vi "Calculator_Calculator-teardown.vi"(10 "Numeric":i32, 11 "test case ID":string) -> (3 "result":bool)   [LabVIEW 2020]
doc: "The teardown VI should be executed after the VI under test in the harness VI. In this VI you can evaluate the outputs of the VI under test.\n\nSee the Help Document for more information. (<b>Help</b> > <b>InstaCoverage Help...</b>)"
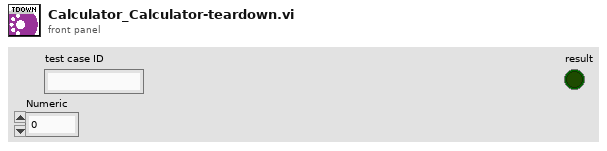
[diagram p1: front panel]
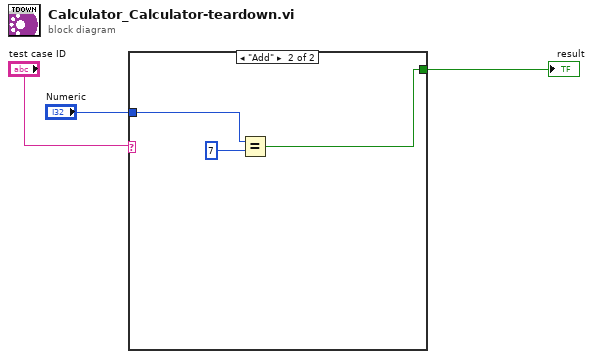
[diagram p0: block diagram]
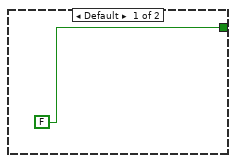
[diagram p2: hidden frame]
diagram:
  n1 = case shown="\"Add\"" "test case ID" {
    tunnel: [FALSE ("result") w7] -> w2
    tunnel: "Numeric" -> [_ w5]
    frame Default {
    }
    frame "Add" {
      n2 = Equal?(x=w5, y=7) -> (x = y?=w7:bool)
    }
  }
  "result" <- w2
